vi "DAQ_E_mIO_DIO.ProcCases.vi"(0 "i ref in":refnum<vi>, 1 "selector":string, 2 "Data":T1, 3 "call cluster":T2={"Object"="", "Selector"="", "CallType"=enum."synchronous", "Async Object"="", "Async Selector"="", "Data Descriptor"="", "Data"=[], "Error #"=0, "Expire"=0}, 5 "error in (no error)":errorcluster) -> (14 "i ref out":refnum<vi>, 17 "answer cluster":T2={"Object"="", "Selector"="", "CallType"=enum."synchronous", "Async Object"="", "Async Selector"="", "Data Descriptor"="", "Data"=[], "Error #"=0, "Expire"=0}, 19 "error out":errorcluster)   [LabVIEW 2014, in "DAQ_E_mIO_DIO.lvlib"]
doc: "This method is called by a process from within the default case in the event loop. The methods of a class that are linked to events will be called from THIS method. Add your code here."
uses:
  DAQ_E_mIO_DIO.lvlib
  CS_Core/CSSystem/CoreDefs/CoreDefs.call_type.ctl
  CS_Core/BaseProcess/BaseProcess.descriptor string definition.ctl
  CS_Core/CSSystem/CoreDefs/CoreDefs.rawDataType.ctl
  CS_Core/CSSystem/CoreLib/CoreLib.string 2 byte array.vi
  CS_Core/CSSystem/CoreLib/CoreLib.int 2 byte array.vi
  CS_Core/CSSystem/CoreLib/CoreLib.byte array 2 int.vi
  CS_Core/CSSystem/CoreLib/CoreLib.short 2 byte array.vi
  CS_Core/CSSystem/CoreLib/CoreLib.byte array 2 short.vi
  CS_Core/CSSystem/CoreLib/CoreLib.lvlib
  CS_Core/BaseProcess/BaseProcess.lvlib
  CS_Core/CSApplicationBaseClasses/DigiIOBase/DigiIOBase.lvlib
  CS_Core/CSApplicationBaseClasses/DeviceBase/DeviceBase.lvlib
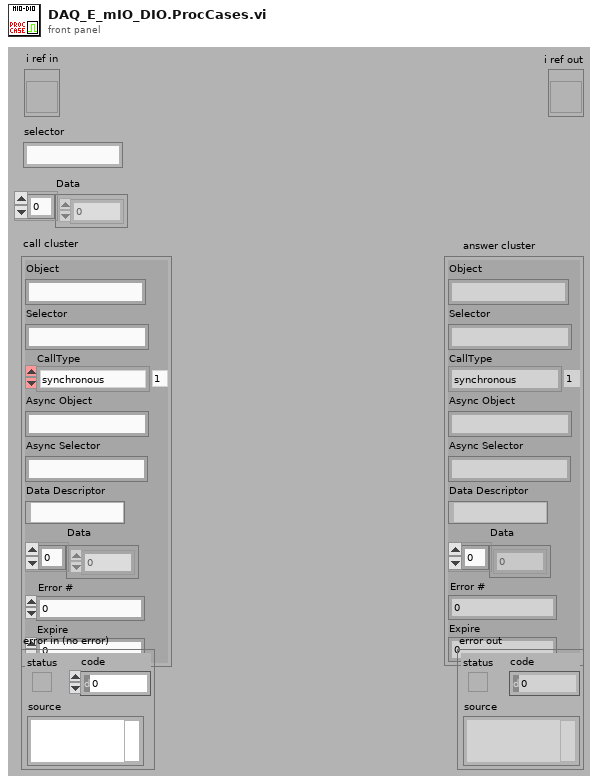
[diagram p1: front panel]
types:
  T1 = typedef "CoreDefs.rawDataType.ctl" = i8[]
  T2 = typedef "CoreDefs.call_type.ctl" = cluster{"Object":string, "Selector":string, "CallType":enum16{"simple", "synchronous", "asynchronous"}, "Async Object":string, "Async Selector":string, "Data Descriptor":T3, "Data":T1, "Error #":i32, "Expire":u32}
  T3 = typedef "BaseProcess.lvlib/BaseProcess.descriptor string definition.ctl" = string
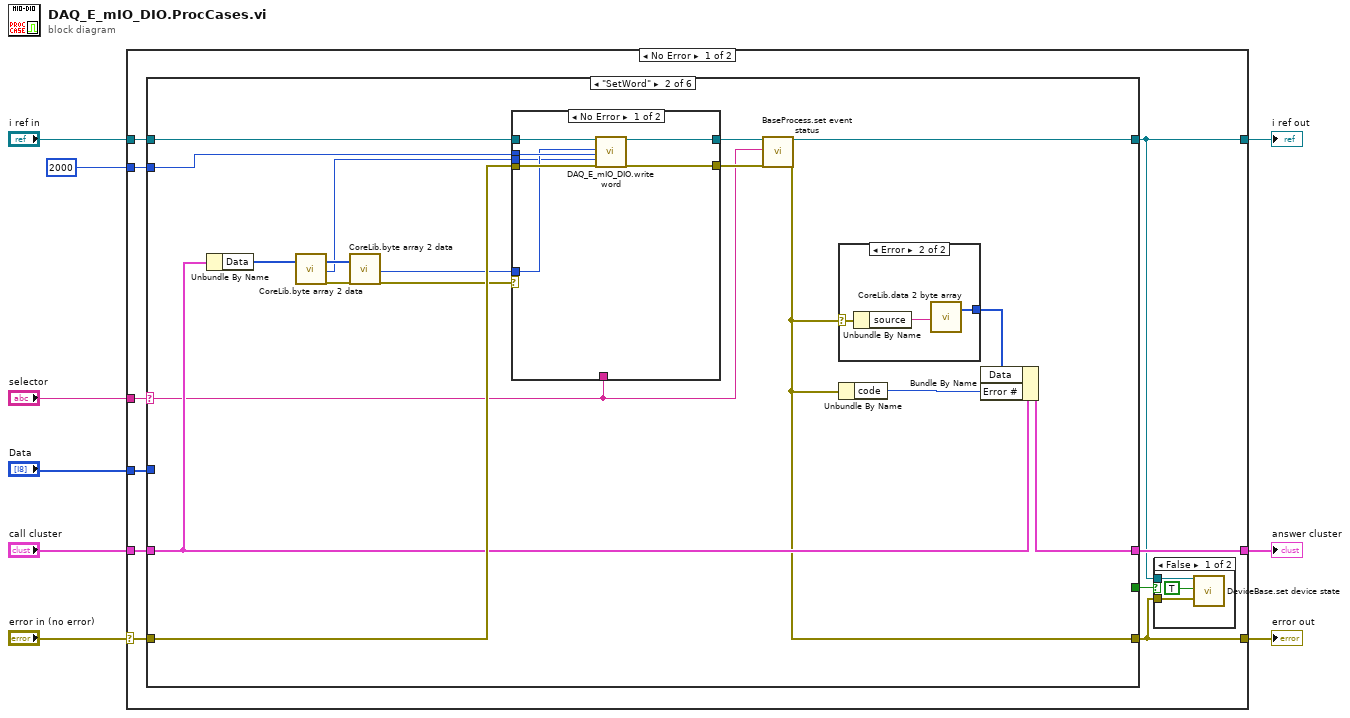
[diagram p0: block diagram]
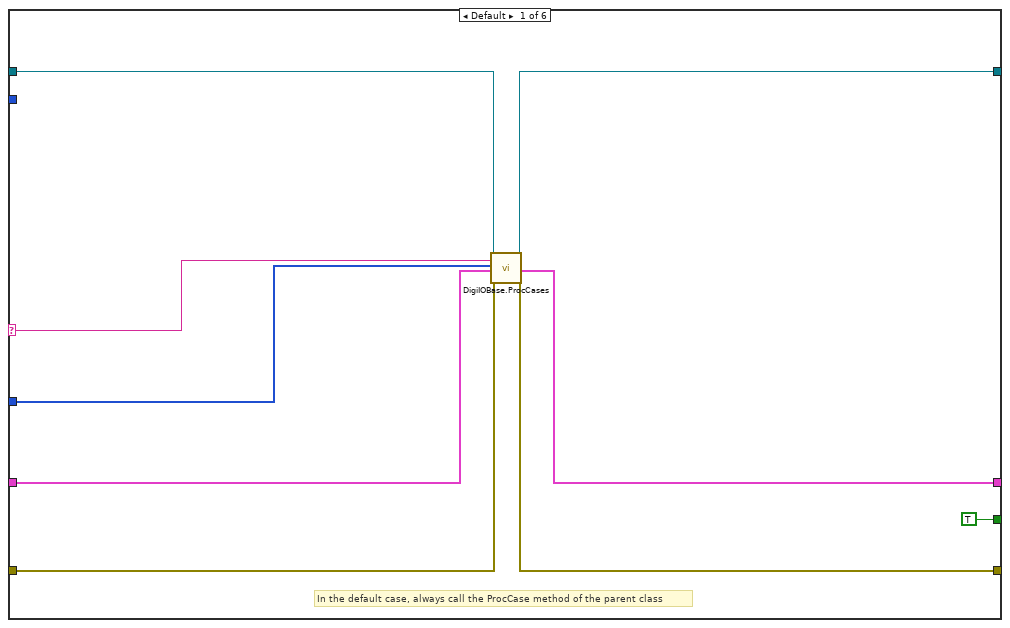
[diagram p3: hidden frame]
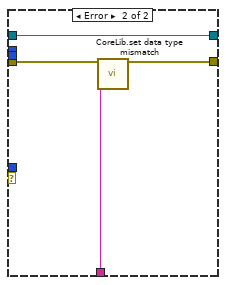
[diagram p5: hidden frame]
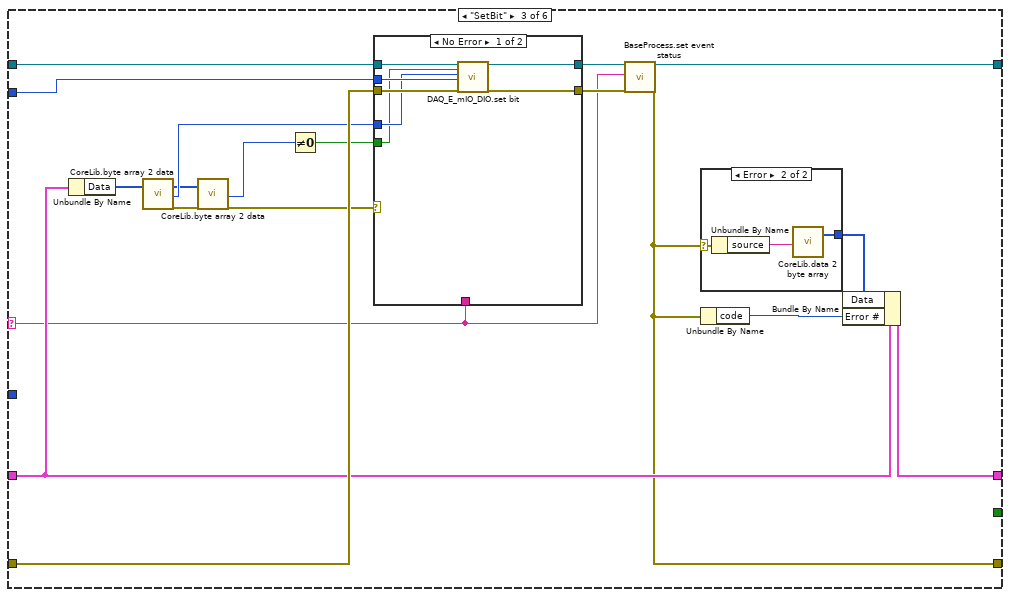
[diagram p6: hidden frame]
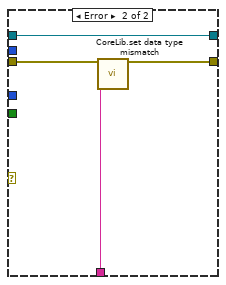
[diagram p8: hidden frame]
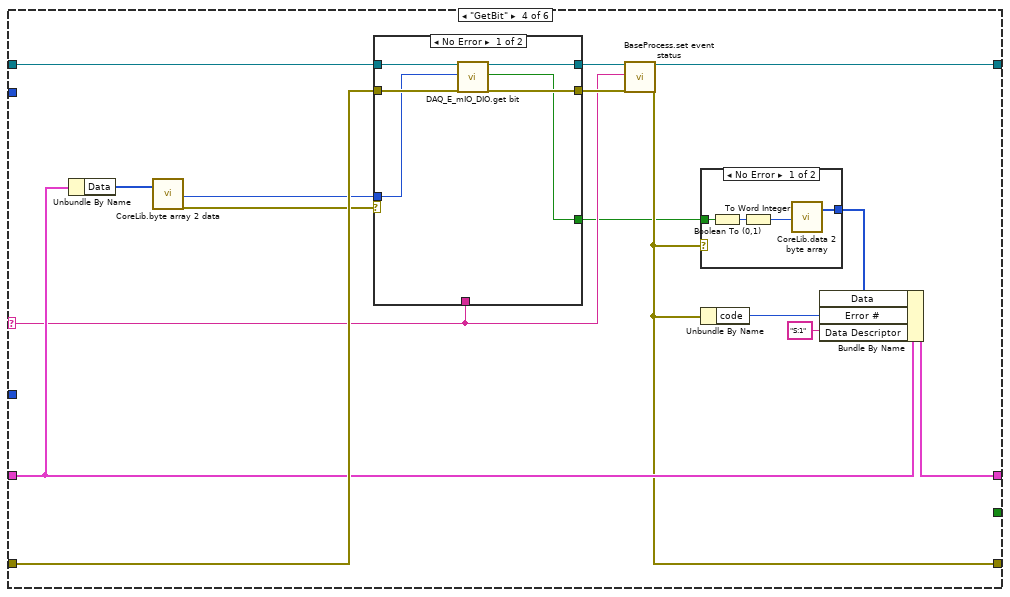
[diagram p9: hidden frame]
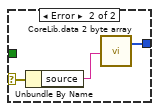
[diagram p10: hidden frame]
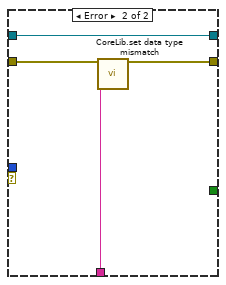
[diagram p11: hidden frame]
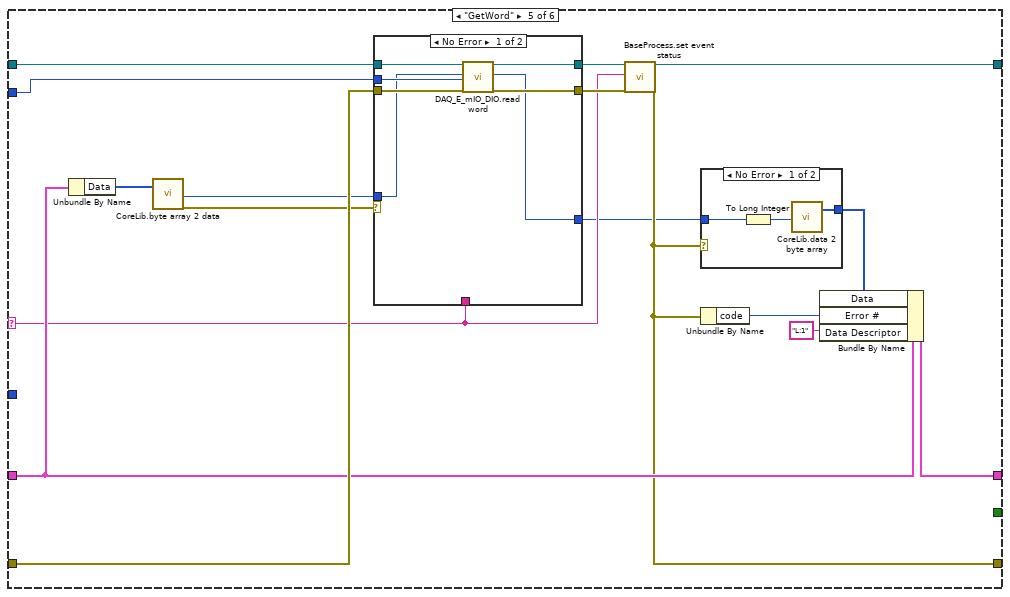
[diagram p12: hidden frame]
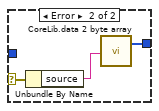
[diagram p13: hidden frame]
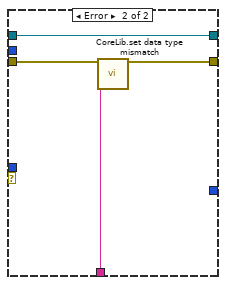
[diagram p14: hidden frame]
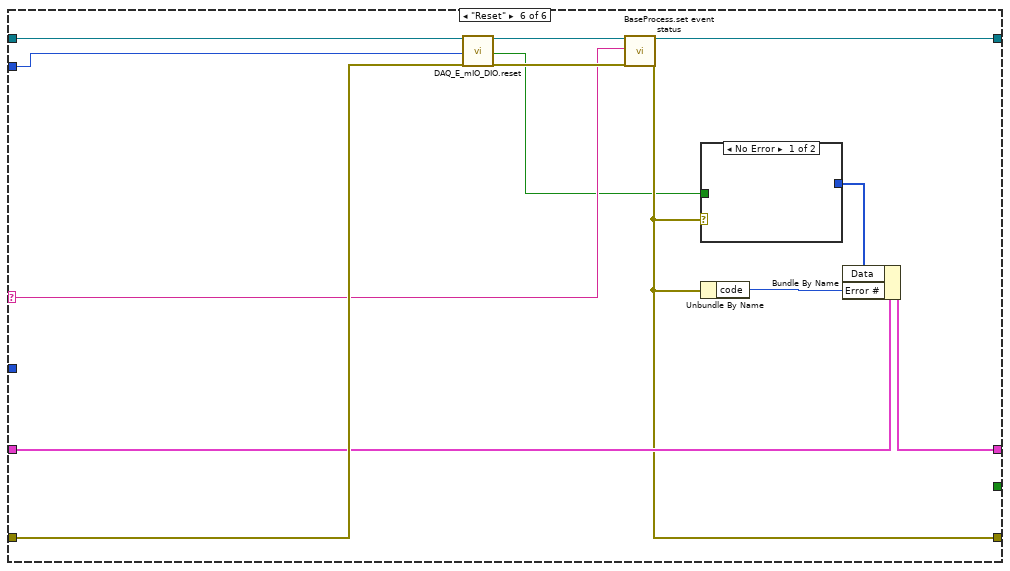
[diagram p15: hidden frame]
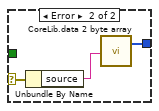
[diagram p16: hidden frame]
diagram:
  n1 = case shown="No Error" "error in (no error)" {
    selector: "error in (no error)" -> [w13 w180]
    tunnel: "selector" -> [w19 _]
    tunnel: [w18 w181] -> w8
    tunnel: "Data" -> [w17 _]
    tunnel: "call cluster" -> [w16 w181]
    tunnel: "i ref in" -> [w15 w182]
    tunnel: [w11 w182] -> w4
    tunnel: [w10 w180] -> w3
    tunnel: 2000 ("ms timeout (10000)") -> [w14 _]
    frame No Error {
      n2 = case shown="\"SetWord\"" w19 {
        selector: w19 -> [w25 w40 w73 w103 w137 w167]
        tunnel: w17 -> [w26 _ _ _ _ _]
        tunnel: w15 -> [w24 w49 w82 w112 w146 w176]
        tunnel: [w31 w39 w72 w102 w136 w166] -> w11
        tunnel: w16 -> [w27 w46 w79 w109 w143 w173]
        tunnel: [w28 w45 w78 w108 w142 w172] -> w18
        tunnel: w13 -> [w30 w48 w81 w111 w145 w175]
        tunnel: [w29 w41 w74 w104 w138 w168] -> w10
        tunnel: w14 -> [_ w38 w71 _ w130 w164]
        tunnel: [TRUE _ _ _ _ _] -> w12
        frame Default {
          # "In the default case, always call the ProcCase method of the parent class"
          n3 = call "DigiIOBase.ProcCases.vi"("i ref in"=w24, "selector"=w25, "Data"=w26, "call cluster"=w27, "error in (no error)"=w30) -> ("i ref out"=w31:refnum<vi>, "answer cluster"=w28:T2, "error out"=w29:errorcluster)  [unwired: 12 in]
        }
        frame "SetWord" {
          n4 = Unbundle By Name(w46) -> ("Data"=w33:T1)
          n5 = call-poly "CoreLib.byte array 2 data.vi"("byteArray"=w33) -> ("byteArray out"=w35:T1, "i32"=w32:i32, "error out"=w34:errorcluster)  [unwired: 16 in]
          n6 = call-poly "CoreLib.byte array 2 data.vi"("byteArray"=w35, "error in (no error)"=w34) -> ("i32"=w37:i32, "error out"=w36:errorcluster)  [unwired: 15 in, 1 out]
          n7 = case shown="No Error" w36 {
            tunnel: [w57 w63] -> w43
            tunnel: w49 -> [w59 w63]
            tunnel: w48 -> [w58 w62]
            tunnel: [w56 w61] -> w42
            tunnel: w40 -> [_ w60]
            tunnel: w37 -> [w54 _]
            tunnel: w38 -> [w55 _]
            tunnel: w32 -> [w53 _]
            frame No Error {
              n8 = call "DAQ_E_mIO_DIO.write word.vi"("i ref in"=w59, "word"=w54, "ms timeout (10000)"=w55, "wordIndex"=w53, "error in (no error)"=w58) -> ("i ref out"=w57:refnum<vi>, "error out"=w56:errorcluster)  [unwired: 12 in, 1 out]
            }
            frame Error {
              n9 = call "CoreLib.set data type mismatch.vi"("error in (no error)"=w62, "error source"=w60) -> ("error out"=w61:errorcluster)  [unwired: 17 in]
            }
          }
          n10 = call "BaseProcess.set event status.vi"("i ref in"=w43, "EventStatus"=w40, "error in (no error)"=w42) -> ("i ref out"=w39:refnum<vi>, "error out"=w41:errorcluster)  [unwired: 14 in, 1 out]
          n11 = case shown="Error" w41 {
            selector: w41 -> [_ w52]
            tunnel: [_ w50] -> w44
            frame No Error {
            }
            frame Error {
              n12 = Unbundle By Name(w52) -> ("source"=w51:string)
              n13 = call-poly "CoreLib.data 2 byte array.vi"("string"=w51) -> ("byteArray out"=w50:T1)  [unwired: 18 in]
            }
          }
          n14 = Unbundle By Name(w41) -> ("code"=w47:i32)
          n15 = Bundle By Name(cluster=w46, "Data"=w44, "Error #"=w47) -> (w45:T2)
        }
        frame "SetBit" {
          n16 = Unbundle By Name(w79) -> ("Data"=w70:T1)
          n17 = call-poly "CoreLib.byte array 2 data.vi"("byteArray"=w70) -> ("byteArray out"=w68:T1, "i32"=w69:i32, "error out"=w67:errorcluster)  [unwired: 16 in]
          n18 = call-poly "CoreLib.byte array 2 data.vi"("byteArray"=w68, "error in (no error)"=w67) -> ("i16"=w65:i16, "error out"=w66:errorcluster)  [unwired: 15 in, 1 out]
          n19 = Not Equal To 0?(x=w65) -> (x != 0?=w64:bool)
          n20 = case shown="No Error" w66 {
            tunnel: [w90 w96] -> w76
            tunnel: w82 -> [w92 w96]
            tunnel: w81 -> [w91 w95]
            tunnel: [w89 w94] -> w75
            tunnel: w73 -> [_ w93]
            tunnel: w69 -> [w87 _]
            tunnel: w71 -> [w88 _]
            tunnel: w64 -> [w86 _]
            frame No Error {
              n21 = call "DAQ_E_mIO_DIO.set bit.vi"("i ref in"=w92, "bit"=w86, "bitNo"=w87, "ms timeout (10000)"=w88, "error in (no error)"=w91) -> ("i ref out"=w90:refnum<vi>, "error out"=w89:errorcluster)  [unwired: 12 in, 1 out]
            }
            frame Error {
              n22 = call "CoreLib.set data type mismatch.vi"("error in (no error)"=w95, "error source"=w93) -> ("error out"=w94:errorcluster)  [unwired: 17 in]
            }
          }
          n23 = call "BaseProcess.set event status.vi"("i ref in"=w76, "EventStatus"=w73, "error in (no error)"=w75) -> ("i ref out"=w72:refnum<vi>, "error out"=w74:errorcluster)  [unwired: 14 in, 1 out]
          n24 = case shown="Error" w74 {
            selector: w74 -> [_ w85]
            tunnel: [_ w83] -> w77
            frame No Error {
            }
            frame Error {
              n25 = Unbundle By Name(w85) -> ("source"=w84:string)
              n26 = call-poly "CoreLib.data 2 byte array.vi"("string"=w84) -> ("byteArray out"=w83:T1)  [unwired: 18 in]
            }
          }
          n27 = Unbundle By Name(w74) -> ("code"=w80:i32)
          n28 = Bundle By Name(cluster=w79, "Data"=w77, "Error #"=w80) -> (w78:T2)
        }
        frame "GetBit" {
          n29 = Unbundle By Name(w109) -> ("Data"=w100:T1)
          n30 = call-poly "CoreLib.byte array 2 data.vi"("byteArray"=w100) -> ("i32"=w99:i32, "error out"=w98:errorcluster)  [unwired: 16 in, 1 out]
          n31 = case shown="No Error" w98 {
            tunnel: [w123 w129] -> w106
            tunnel: w112 -> [w125 w129]
            tunnel: w111 -> [w124 w128]
            tunnel: [w122 w127] -> w105
            tunnel: w103 -> [_ w126]
            tunnel: w99 -> [w121 _]
            tunnel: [w120 _] -> w101
            frame No Error {
              n32 = call "DAQ_E_mIO_DIO.get bit.vi"("i ref in"=w125, "bitIndex"=w121, "error in (no error)"=w124) -> ("i ref out"=w123:refnum<vi>, "bit"=w120:bool, "error out"=w122:errorcluster)  [unwired: 13 in, 1 out]
            }
            frame Error {
              n33 = call "CoreLib.set data type mismatch.vi"("error in (no error)"=w128, "error source"=w126) -> ("error out"=w127:errorcluster)  [unwired: 17 in]
            }
          }
          n34 = call "BaseProcess.set event status.vi"("i ref in"=w106, "EventStatus"=w103, "error in (no error)"=w105) -> ("i ref out"=w102:refnum<vi>, "error out"=w104:errorcluster)  [unwired: 14 in, 1 out]
          n35 = case shown="No Error" w104 {
            selector: w104 -> [_ w119]
            tunnel: [w113 w117] -> w107
            tunnel: w101 -> [w116 _]
            frame No Error {
              n36 = Boolean To (0,1)(Boolean=w116) -> (0, 1=w115:i16)
              n37 = To Word Integer(number=w115) -> (16bit integer=w114:i16)
              n38 = call-poly "CoreLib.data 2 byte array.vi"("i16"=w114) -> ("byteArray out"=w113:T1)  [unwired: 18 in]
            }
            frame Error {
              n39 = Unbundle By Name(w119) -> ("source"=w118:string)
              n40 = call-poly "CoreLib.data 2 byte array.vi"("string"=w118) -> ("byteArray out"=w117:T1)  [unwired: 18 in]
            }
          }
          n41 = Unbundle By Name(w104) -> ("code"=w110:i32)
          n42 = Bundle By Name(cluster=w109, "Data"=w107, "Error #"=w110, "Data Descriptor"="S:1") -> (w108:T2)
        }
        frame "GetWord" {
          n43 = Unbundle By Name(w143) -> ("Data"=w134:T1)
          n44 = call-poly "CoreLib.byte array 2 data.vi"("byteArray"=w134) -> ("i32"=w133:i32, "error out"=w132:errorcluster)  [unwired: 16 in, 1 out]
          n45 = case shown="No Error" w132 {
            tunnel: [w155 w163] -> w140
            tunnel: w146 -> [w159 w163]
            tunnel: w145 -> [w158 w162]
            tunnel: [w154 w161] -> w139
            tunnel: w137 -> [_ w160]
            tunnel: w133 -> [w156 _]
            tunnel: [w153 _] -> w135
            tunnel: w130 -> [w157 _]
            frame No Error {
              n46 = call "DAQ_E_mIO_DIO.read word.vi"("i ref in"=w159, "wordIndex"=w156, "ms timeout (10000)"=w157, "error in (no error)"=w158) -> ("i ref out"=w155:refnum<vi>, "word"=w153:u8, "error out"=w154:errorcluster)  [unwired: 12 in, 1 out]
            }
            frame Error {
              n47 = call "CoreLib.set data type mismatch.vi"("error in (no error)"=w162, "error source"=w160) -> ("error out"=w161:errorcluster)  [unwired: 17 in]
            }
          }
          n48 = call "BaseProcess.set event status.vi"("i ref in"=w140, "EventStatus"=w137, "error in (no error)"=w139) -> ("i ref out"=w136:refnum<vi>, "error out"=w138:errorcluster)  [unwired: 14 in, 1 out]
          n49 = case shown="No Error" w138 {
            selector: w138 -> [_ w152]
            tunnel: [w148 w150] -> w141
            tunnel: w135 -> [w147 _]
            frame No Error {
              n50 = To Long Integer(number=w147) -> (32bit integer=w149:i32)
              n51 = call-poly "CoreLib.data 2 byte array.vi"("i32"=w149) -> ("byteArray out"=w148:T1)  [unwired: 18 in]
            }
            frame Error {
              n52 = Unbundle By Name(w152) -> ("source"=w151:string)
              n53 = call-poly "CoreLib.data 2 byte array.vi"("string"=w151) -> ("byteArray out"=w150:T1)  [unwired: 18 in]
            }
          }
          n54 = Unbundle By Name(w138) -> ("code"=w144:i32)
          n55 = Bundle By Name(cluster=w143, "Data"=w141, "Error #"=w144, "Data Descriptor"="L:1") -> (w142:T2)
        }
        frame "Reset" {
          n56 = call "DAQ_E_mIO_DIO.reset.vi"("i ref in"=w176, "ms timeout (10000)"=w164, "error in (no error)"=w175) -> ("i ref out"=w170:refnum<vi>, "timed out"=w165:bool, "error out"=w169:errorcluster)  [unwired: 14 in]
          n57 = call "BaseProcess.set event status.vi"("i ref in"=w170, "EventStatus"=w167, "error in (no error)"=w169) -> ("i ref out"=w166:refnum<vi>, "error out"=w168:errorcluster)  [unwired: 14 in, 1 out]
          n58 = case shown="No Error" w168 {
            selector: w168 -> [_ w179]
            tunnel: [_ w177] -> w171
            tunnel: w165 -> [_ _]
            frame No Error {
            }
            frame Error {
              n59 = Unbundle By Name(w179) -> ("source"=w178:string)
              n60 = call-poly "CoreLib.data 2 byte array.vi"("string"=w178) -> ("byteArray out"=w177:T1)  [unwired: 18 in]
            }
          }
          n61 = Unbundle By Name(w168) -> ("code"=w174:i32)
          n62 = Bundle By Name(cluster=w173, "Data"=w171, "Error #"=w174) -> (w172:T2)
        }
      }
      n63 = case shown="False" w12 {
        tunnel: w11 -> [w21 _]
        tunnel: w10 -> [w20 _]
        frame False {
          n64 = call "DeviceBase.set device state.vi"("i ref in"=w21, "implicit"=TRUE, "device error"=w20) -> ()  [unwired: 14 in, 3 out]
        }
        frame True {
        }
      }
    }
    frame Error {
    }
  }
  "answer cluster" <- w8
  "i ref out" <- w4
  "error out" <- w3
